vi "Sample Transfer Set Containers for Purging.vi"(8 "error in (no error)":errorcluster, 11 "cRIO-CO2 in":refnum<class "cRIO-CO2.lvclass">) -> (0 "error out":errorcluster, 3 "cRIO-CO2 out":refnum<class "cRIO-CO2.lvclass">)   [LabVIEW 2015, in "cRIO-Carbondioxide.lvlib" / "cRIO-CO2.lvlib" / "cRIO-CO2.lvclass"]
uses:
  cRIO-CO2.lvclass
  cRIO-CO2.lvclass/cRIO-CO2.ctl
  Sample Line Messages/Open Line Msg/Open Line Msg.lvclass/Open Line Msg.ctl
  <vilib>/ActorFramework/Message Enqueuer/Message Enqueuer.lvclass/Message Enqueuer.ctl
  Controls/Sample Transfer Container Enumerator.ctl
  Storage Line Messages/Set Line Msg/Set Line Msg.lvclass/Set Line Msg.ctl
  Syringe Line Messages/Set Syringe Valve/Set Valve Msg/Set Syringe Valve Msg.lvclass/Set Syringe Valve Msg.ctl
  <vilib>/ActorFramework/Message Enqueuer/Enqueue.vi
  <vilib>/ActorFramework/Message Priority Queue/Priority Enqueue.vi
  Interlocks/Interlock Chain/Interlock Chain.lvclass
  Sample Line Messages/Open Line Msg/Open Line Msg.lvclass
  Storage Line Messages/Set Line Msg/Set Line Msg.lvclass
  Syringe Line Messages/Set Syringe Valve/Set Valve Msg/Set Syringe Valve Msg.lvclass
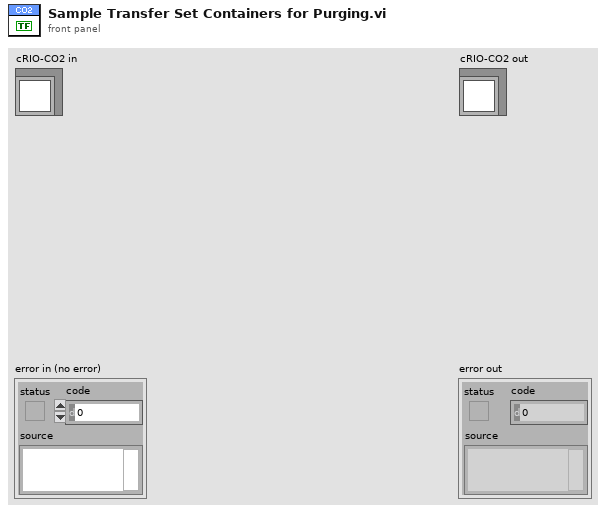
[diagram p1: front panel]
types:
  T1 = typedef "Sample Transfer Container Enumerator.ctl" = enum16{"None", "Sample 1", "Sample 2", "Sample 3", "Sample 4", "Sample 5", "Storage 01", "Storage 02", "Storage 03", "Storage 04", "Storage 05", "Storage 06", "Storage 07", "Storage 08", "Storage 09", "Storage 10", "Storage 11", "Storage 12", "Syringe", "Undefined"}
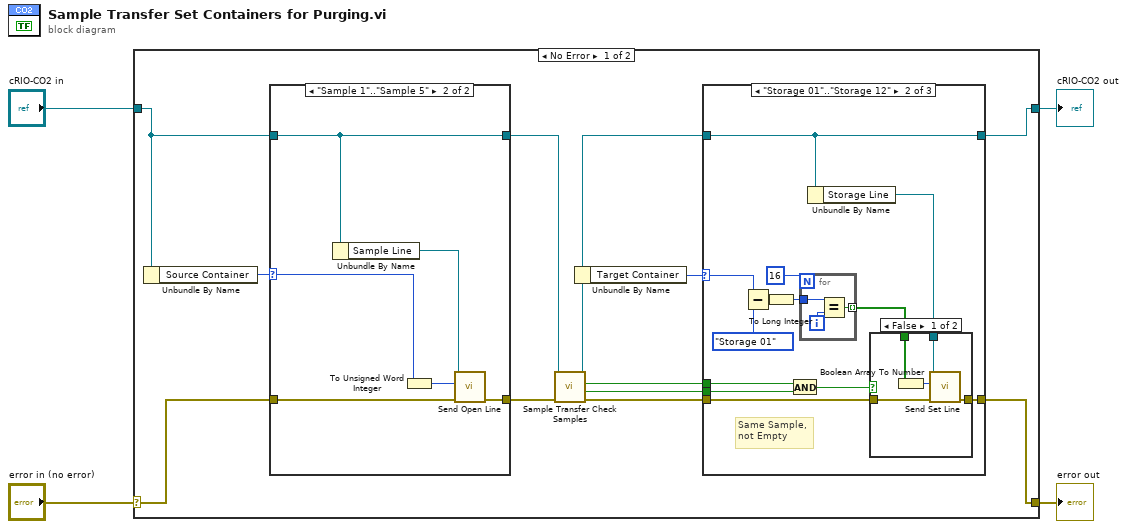
[diagram p0: block diagram]
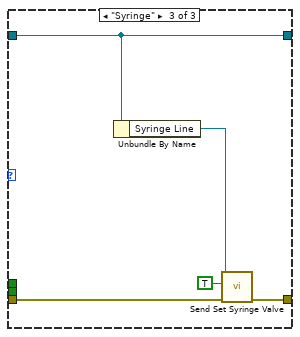
[diagram p4: hidden frame]
diagram:
  n1 = case shown="No Error" "error in (no error)" {
    selector: "error in (no error)" -> [w13 w55]
    tunnel: [w12 w55] -> w3
    tunnel: [w11 w54] -> w1
    tunnel: "cRIO-CO2 in" -> [w14 w54]
    frame No Error {
      n2 = Unbundle By Name(w14) -> ("Source Container"=w16:T1)
      n3 = case shown="\"Sample 1\"..\"Sample 5\"" w16 {
        selector: w16 -> [_ w49]
        tunnel: w13 -> [w46 w52]
        tunnel: w14 -> [w47 w53]
        tunnel: [w47 w53] -> w8
        tunnel: [w46 w51] -> w10
        frame "Undefined", Default {
        }
        frame "Sample 1".."Sample 5" {
          n4 = Unbundle By Name(w53) -> ("Sample Line"=w50:refnum<class "Message Enqueuer.lvclass">)
          n5 = To Unsigned Word Integer(number=w49) -> (unsigned 16bit integer=w48:u16)
          n6 = call "Send Open Line.vi"("error in (no error)"=w52, "Sample Line (All Closed)"=w48, "Message Enqueuer"=w50) -> ("error out"=w51:errorcluster)  [unwired: 7 in, 1 out]
        }
      }
      n7 = call "Sample Transfer Check Samples.vi"("error in (no error)"=w10, "cRIO-CO2 in"=w8) -> ("error out"=w9:errorcluster, "Target not Empty"=w5:bool, "Same Sample in Source and Target"=w6:bool, "cRIO-CO2 out"=w7:refnum<class "cRIO-CO2.lvclass">)  [unwired: 5 in, 1 out]
      n8 = Unbundle By Name(w7) -> ("Target Container"=w15:T1)
      n9 = case shown="\"Storage 01\"..\"Storage 12\"" w15 {
        selector: w15 -> [_ w27 _]
        tunnel: w9 -> [w17 w30 w42]
        tunnel: w7 -> [w18 w31 w43]
        tunnel: [w18 w31 w43] -> w11
        tunnel: [w17 w29 w45] -> w12
        tunnel: w6 -> [_ w21 _]
        tunnel: w5 -> [_ w20 _]
        frame "Undefined", Default {
        }
        frame "Storage 01".."Storage 12" {
          # "Same Sample,\nnot Empty"
          n10 = Subtract(x=w27, y=Sample_Transfer_Container_Enumerator."Storage 01") -> (x-y=w22:u16)
          n11 = To Long Integer(number=w22) -> (32bit integer=w24:i32)
          n12 = And(x=w21, y=w20) -> (x .and. y?=w19:bool)
          n13 = for {
            N: 16 -> [_]
            tunnel: w24 -> [w40]
            tunnel: [w38] -> w23 mode=indexing
            i -> [w39]
            n14 = Equal?(x=w40, y=w39) -> (x = y?=w38:bool)
          }
          n15 = Unbundle By Name(w31) -> ("Storage Line"=w28:refnum<class "Message Enqueuer.lvclass">)
          n16 = case shown="False" w19 {
            tunnel: w30 -> [w36 w37]
            tunnel: [w35 w37] -> w29
            tunnel: w28 -> [w34 _]
            tunnel: w23 -> [w32 _]
            frame False {
              n17 = Boolean Array To Number(Boolean array=w32) -> (number=w33:u32)
              n18 = call "Send Set Line.vi"("error in (no error)"=w36, "Bit Field"=w33, "Message Enqueuer"=w34) -> ("error out"=w35:errorcluster)  [unwired: 7 in, 1 out]
            }
            frame True {
            }
          }
        }
        frame "Syringe" {
          n19 = Unbundle By Name(w43) -> ("Syringe Line"=w44:refnum<class "Message Enqueuer.lvclass">)
          n20 = call "Send Set Syringe Valve.vi"("error in (no error)"=w42, "Open? (False)"=TRUE, "Message Enqueuer"=w44) -> ("error out"=w45:errorcluster)  [unwired: 7 in, 1 out]
        }
      }
    }
    frame Error {
    }
  }
  "error out" <- w3
  "cRIO-CO2 out" <- w1
